vi "Tag initialize.vi"(9 "namespace":string caption="namespace (top-level VI)", 11 "Tag IN":T1={"Tag Name"=["LStatus", "RStatus", "LTargetTemp", "LTemp1", "LTemp2", "LTemp3", "LTemp4", "LTemp5", "LTemp6", "RTargetT", "RTemp1", "RTemp2", "RTemp3", "RTemp4", "RTemp5", "RTemp6", "LWO", "LOPID", "LDate", "LTime", "LModel", "LAgingTime", "LAgingTemp", "LStartTime", "LEndTime", "RWO", "ROPID", "RDate", "RTime", "RModel", "RAgingTime", "RAgingTemp", "RStartTime", "REndTime"], "Tag Type"=[enum."String", enum."String", enum."Double", enum."Double", enum."Double", enum."Double", enum."Double", enum."Double", enum."Double", enum."Double", enum."Double", enum."Double", enum."Double", enum."Double", enum."Double", enum."Double", enum."String", enum."String", enum."String", enum."String", enum."String", enum."String", enum."String", enum."String", enum."String", enum."String", enum."String", enum."String", enum."String", enum."String", enum."String", enum."String", enum."String", enum."String"], "Tag Data"=[], "Skyline Array"=[]}) -> (0 "error out":errorcluster, 3 "output cluster":T1={"Tag Name"=["LStatus", "RStatus", "LTargetTemp", "LTemp1", "LTemp2", "LTemp3", "LTemp4", "LTemp5", "LTemp6", "RTargetT", "RTemp1", "RTemp2", "RTemp3", "RTemp4", "RTemp5", "RTemp6", "LWO", "LOPID", "LDate", "LTime", "LModel", "LAgingTime", "LAgingTemp", "LStartTime", "LEndTime", "RWO", "ROPID", "RDate", "RTime", "RModel", "RAgingTime", "RAgingTemp", "RStartTime", "REndTime"], "Tag Type"=[enum."String", enum."String", enum."Double", enum."Double", enum."Double", enum."Double", enum."Double", enum."Double", enum."Double", enum."Double", enum."Double", enum."Double", enum."Double", enum."Double", enum."Double", enum."Double", enum."String", enum."String", enum."String", enum."String", enum."String", enum."String", enum."String", enum."String", enum."String", enum."String", enum."String", enum."String", enum."String", enum."String", enum."String", enum."String", enum."String", enum."String"], "Tag Data"=[], "Skyline Array"=[]})   [LabVIEW 2017]
uses:
  Tag.ctl
  <vilib>/Skyline/Tag/Shared/typedefs/DataType.ctl
  <vilib>/Skyline/Tag/Wrapper/Wrapper_class/NI Skyline Tag.lvclass
  <vilib>/Skyline/Tag/Wrapper/Wrapper AMQP_class/Open Tag AMQP.vi
  <vilib>/Skyline/Tag/Shared/NI Skyline Tag.lvlib
  <vilib>/Skyline/Tag/Wrapper/Wrapper AMQP_class/NI Skyline Tag AMQP.lvclass
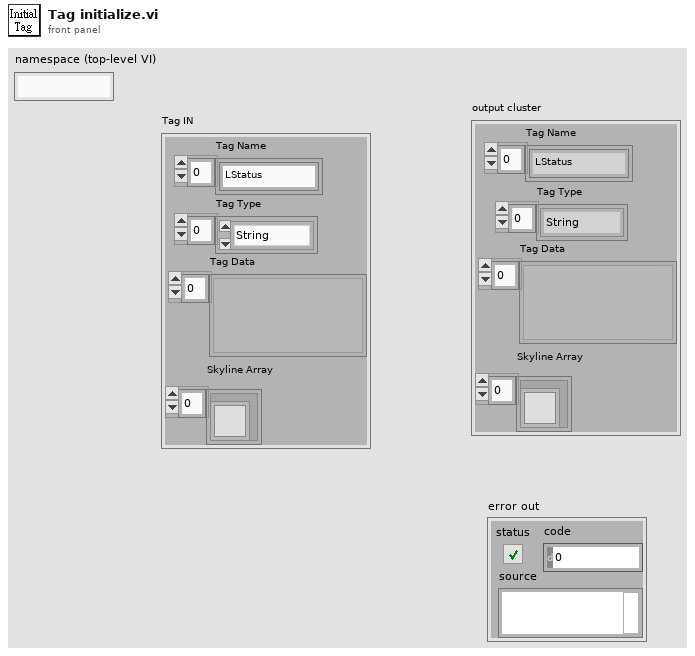
[diagram p1: front panel]
types:
  T1 = typedef "Tag.ctl" = cluster{"Tag Name":string[], "Tag Type":T2[], "Tag Data":variant[], "Skyline Array":refnum<class "NI Skyline Tag.lvclass">[]}
  T2 = typedef "NI Skyline Tag.lvlib/DataType.ctl" = enum32{"Double", "I32", "String", "Boolean", "U64", "Timestamp"}
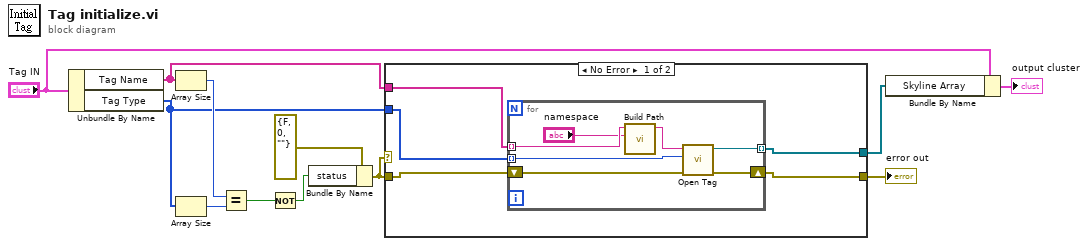
[diagram p0: block diagram]
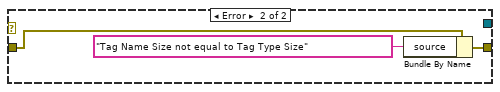
[diagram p2: hidden frame]
diagram:
  n1 = Unbundle By Name("Tag IN") -> ("Tag Name"=w5:string[], "Tag Type"=w6:T2[])
  n2 = Array Size(array=w5) -> (size(s)=w7:i32)
  n3 = Array Size(array=w6) -> (size(s)=w8:i32)
  n4 = Equal?(x=w7, y=w8) -> (x = y?=w10:bool)
  n5 = Not(x=w10) -> (.not. x?=w4:bool)
  n6 = Bundle By Name(cluster=errorcluster {"status"=FALSE, "code"=0, "source"=""} ("error constant"), "status"=w4) -> (w11:errorcluster)
  n7 = case shown="No Error" w11 {
    tunnel: w5 -> [w17 _]
    tunnel: w6 -> [w16 _]
    tunnel: w11 -> [w15 w27]
    tunnel: [w14 w26] -> w12
    tunnel: [w13 _] -> w2
    frame No Error {
      n8 = for {
        tunnel: w17 -> [w23] mode=indexing
        tunnel: w16 -> [w22] mode=indexing
        tunnel: [w21] -> w13 mode=indexing
        shift-right: [w20] -> w14
        shift-left: w15 -> [w19]
        n9 = call <vilib>:"Build Path.vi"("namespace"="namespace", "tag name"=w23) -> ("path"=w24:string)  [unwired: 9 in]
        n10 = call-poly <vilib>:"Open Tag.vi"("error in (no error)"=w19, "data type"=w22, "path"=w24) -> ("error out"=w20:errorcluster, "tag out"=w21:refnum<class "NI Skyline Tag.lvclass">)  [unwired: 7 in]
      }
    }
    frame Error {
      n11 = Bundle By Name(cluster=w27, "source"="Tag Name Size not equal to Tag Type Size") -> (w26:errorcluster)
    }
  }
  "error out" <- w12
  n12 = Bundle By Name(cluster="Tag IN", "Skyline Array"=w2) -> (→"output cluster":T1)
